vi "HeaterConfigurationGlobal.vi"(5 "Index":u16, 7 "Action":T2=enum."Get", 8 "Error In":errorcluster, 11 "Set Value":T1={"VISA Resource"="", "COM Port"=1, "Setpoint"=0.0, "Standby?"=FALSE}) -> (0 "Error Out":errorcluster, 2 "Heater Count":i32, 3 "Value Out":T1={"VISA Resource"="", "COM Port"=1, "Setpoint"=0.0, "Standby?"=FALSE})   [LabVIEW 2012]
uses:
  HeaterConfigurationGlobalAction.ctl
  HeaterConfiguration.ctl
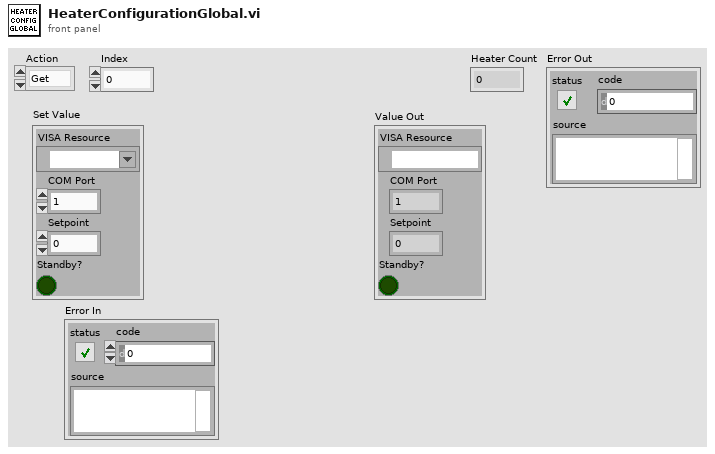
[diagram p1: front panel]
types:
  T1 = typedef "HeaterConfiguration.ctl" = cluster{"VISA Resource":refnum<visa-resource-name>, "COM Port":u8, "Setpoint":dbl, "Standby?":bool}
  T2 = typedef "HeaterConfigurationGlobalAction.ctl" = enum16{"Init", "Get", "Set", "Add", "Remove", "Reset"}
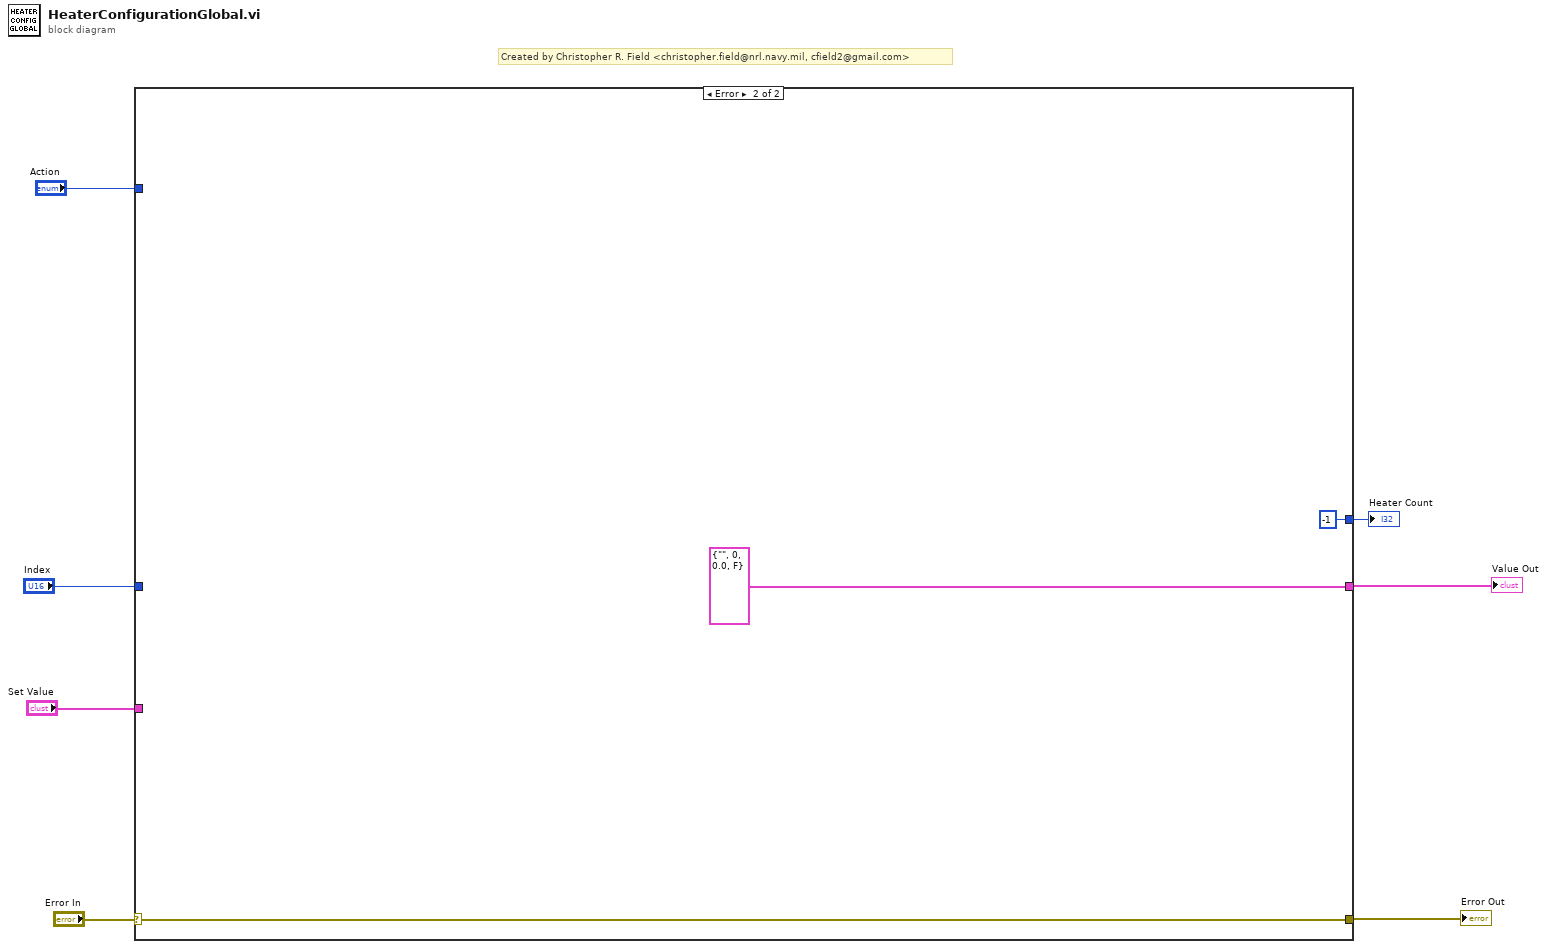
[diagram p0: block diagram]
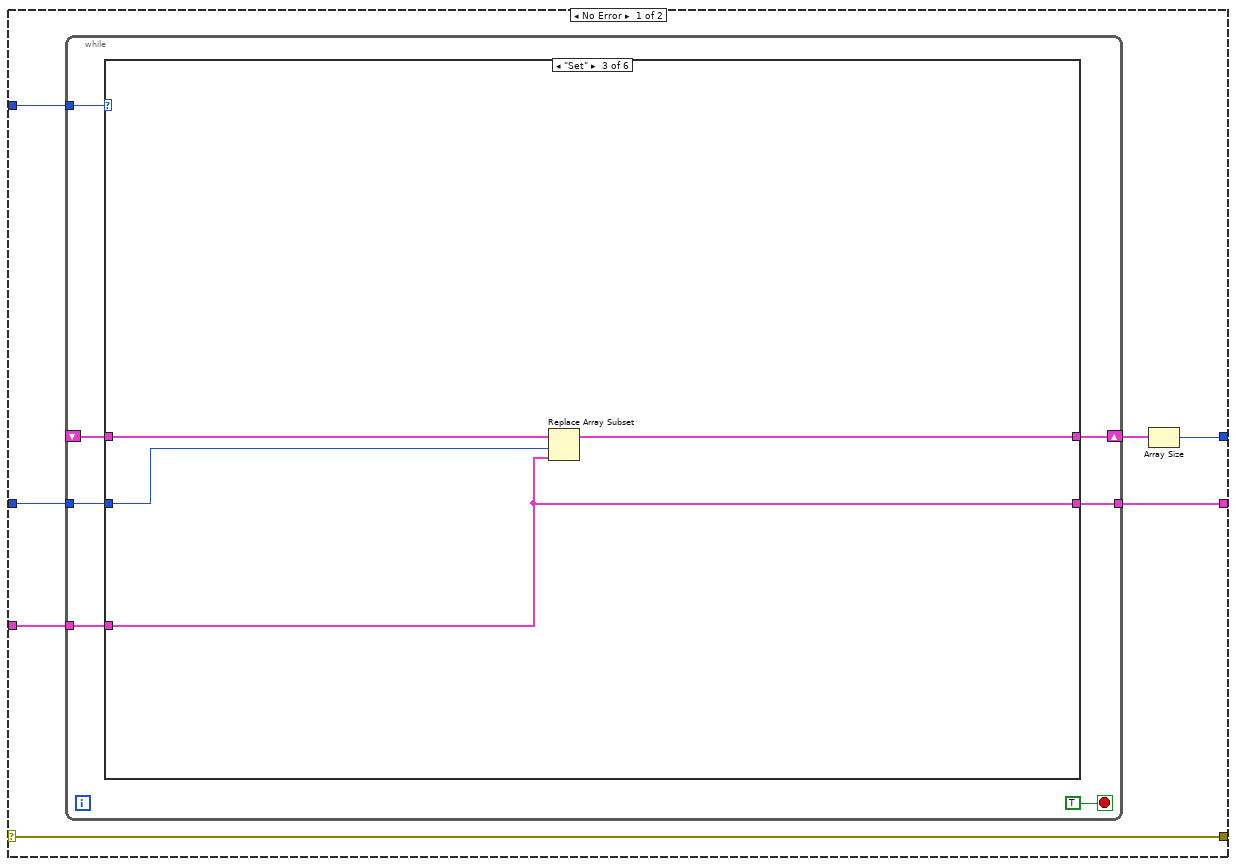
[diagram p2: hidden frame]
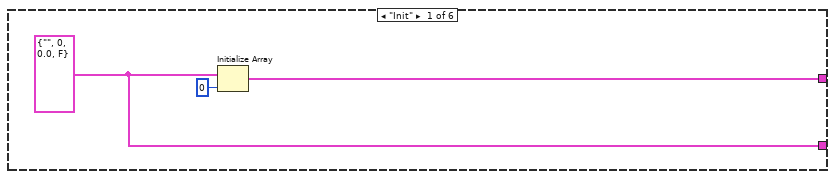
[diagram p3: hidden frame]
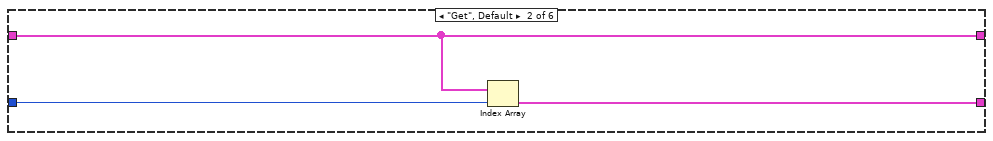
[diagram p4: hidden frame]
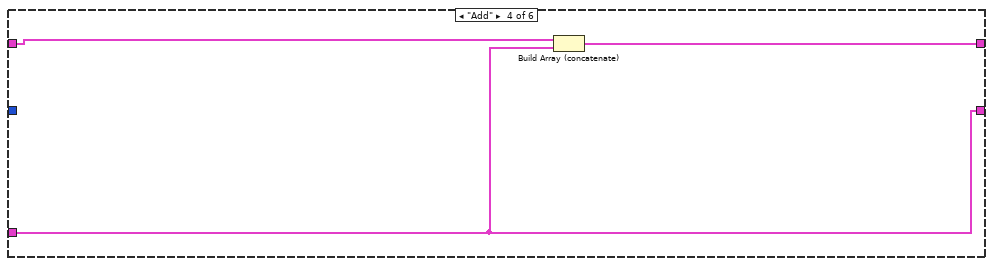
[diagram p5: hidden frame]
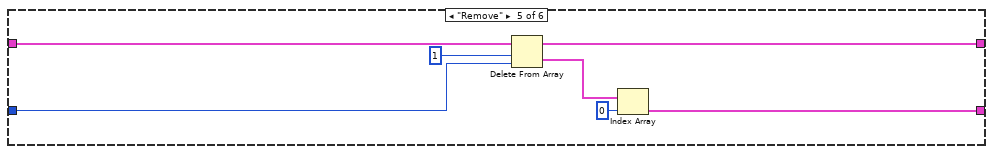
[diagram p6: hidden frame]
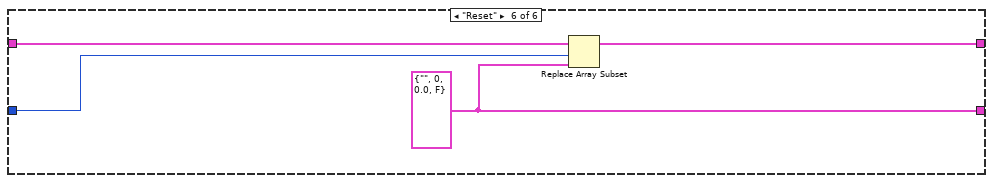
[diagram p7: hidden frame]
diagram:
  # "Created by Christopher R. Field <christopher.field@nrl.navy.mil, cfield2@gmail.com>"
  n1 = case shown="Error" "Error In" {
    selector: "Error In" -> [w10 w47]
    tunnel: "Action" -> [w14 _]
    tunnel: "Set Value" -> [w13 _]
    tunnel: "Index" -> [w12 _]
    tunnel: [w11 T1 {"VISA Resource"="", "COM Port"=0, "Setpoint"=0.0, "Standby?"=FALSE} ("Set Value")] -> w4
    tunnel: [w10 w47] -> w2
    tunnel: [w8 -1] -> w1
    frame No Error {
      n2 = while {
        tunnel: w14 -> [w20]
        tunnel: w13 -> [w19]
        shift-right: [w18] -> w9
        shift-left: _ -> [w17]
        tunnel: w12 -> [w16]
        tunnel: [w15] -> w11
        stop <- TRUE stop-if-true
        n3 = case shown="\"Set\"" w20 {
          tunnel: w19 -> [_ _ w28 w32 _ _]
          tunnel: [w23 w27 w30 w34 w38 w43] -> w18
          tunnel: w17 -> [_ w27 w31 w33 w41 w45]
          tunnel: w16 -> [_ w26 w29 _ w39 w44]
          tunnel: [w22 w25 w28 w32 w35 w42] -> w15
          frame "Init" {
            w22 = T1 {"VISA Resource"="", "COM Port"=0, "Setpoint"=0.0, "Standby?"=FALSE} ("Set Value")
            n4 = Initialize Array(w22, 0 ("dimension size")) -> (w23:T1[])
          }
          frame "Get", Default {
            n5 = Index Array(array=w27, index=w26) -> (element=w25:T1)
          }
          frame "Set" {
            n6 = Replace Array Subset(array=w31, new element=w28, index=w29) -> (w30:T1[])
          }
          frame "Add" {
            n7 = Build Array (concatenate)(w33, w32) -> (w34:T1[])
          }
          frame "Remove" {
            n8 = Delete From Array(array=w41, length=1, index=w39) -> (deleted portion=w37:T1[], array with subset deleted=w38:T1[])
            n9 = Index Array(array=w37, index=0) -> (element=w35:T1)
          }
          frame "Reset" {
            w42 = T1 {"VISA Resource"="", "COM Port"=0, "Setpoint"=0.0, "Standby?"=FALSE} ("Set Value")
            n10 = Replace Array Subset(array=w45, new element=w42, index=w44) -> (w43:T1[])
          }
        }
      }
      n11 = Array Size(array=w9) -> (size(s)=w8:i32)
    }
    frame Error {
    }
  }
  "Value Out" <- w4
  "Error Out" <- w2
  "Heater Count" <- w1
